vi "Start App.vi"(8 "error in (no error)":errorcluster, 11 "VolatusCore in":refnum<class "VolatusCore.lvclass">) -> (0 "error out":errorcluster, 3 "VolatusCore out":refnum<class "VolatusCore.lvclass">)   [LabVIEW 2020, in "Volatus.lvlib" / "VolatusCore.lvclass"]
uses:
  VolatusCore.lvclass
  VolatusCore.lvclass/VolatusCore.ctl
  App/App.lvclass
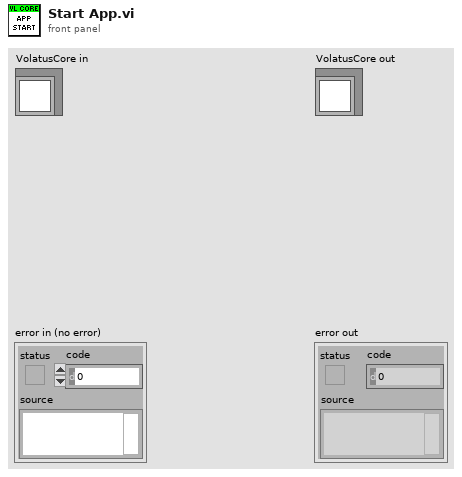
[diagram p1: front panel]
types:
  T1 = typedef "Volatus.lvlib/Core APIs.ctl" = cluster{"Volatus":refnum<class "VolatusAPI.lvclass">, "Event":refnum<class "EventAPI.lvclass">, "Config":refnum<class "ConfigAPI.lvclass">}
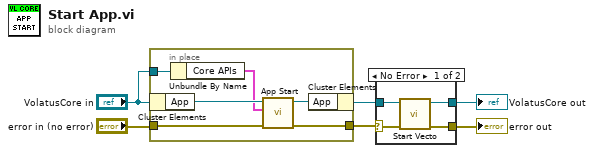
[diagram p0: block diagram]
diagram:
  n1 = in-place {
    in-place-border: "error in (no error)" -> [w12]
    in-place-border: [w11] -> w3
    in-place-border: "VolatusCore in" -> [w9]
    n2 = in-place-cluster #1("VolatusCore in") -> ("App"=w10:refnum<class "App.lvclass">)
    n3 = Unbundle By Name(w9) -> ("Core APIs"=w8:T1)
    n4 = call-dynamic "App Start.vi"("error in (no error)"=w12, "Core APIs"=w8, "App in"=w10) -> ("error out"=w11:errorcluster, "App out"=w7:refnum<class "App.lvclass">)  [unwired: 7 in]
    n5 = in-place-cluster #1("App"=w7) -> (w4:refnum<class "VolatusCore.lvclass">)
  }
  n6 = case shown="No Error" w3 {
    selector: w3 -> [w16 w17]
    tunnel: [w15 w17] -> w2
    tunnel: w4 -> [w14 w18]
    tunnel: [w13 w18] -> w1
    frame No Error {
      n7 = call "Start Vecto.vi"("error in (no error)"=w16, "VolatusCore in"=w14) -> ("error out"=w15:errorcluster, "VolatusCore out"=w13:refnum<class "VolatusCore.lvclass">)  [unwired: 8 in]
    }
    frame Error {
    }
  }
  "error out" <- w2
  "VolatusCore out" <- w1
